vi "acquisitionZProjection.vi"(1 "axis (z)":u16(ring)=2 items=["x", "y", "z"], 2 "z stack":u16[][][](array[numeric])) -> (0 "projected img":u32[][](array[numeric]))   [LabVIEW 2017]
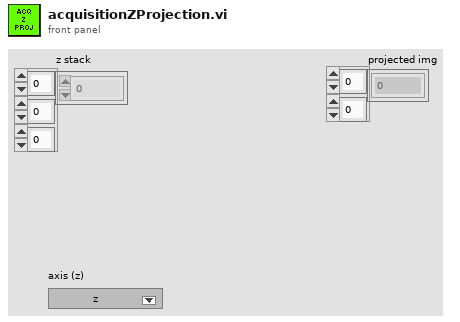
[diagram p1: front panel]
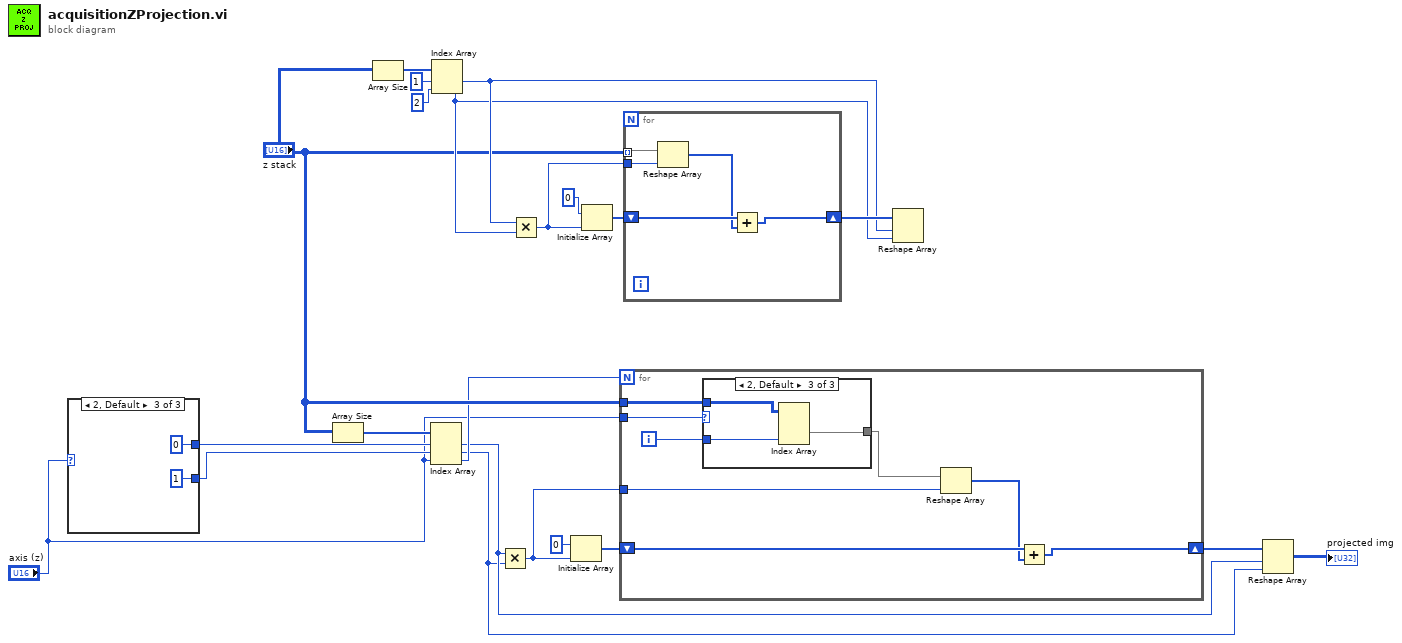
[diagram p0: block diagram]
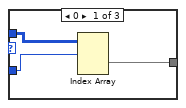
[diagram p2: hidden frame]
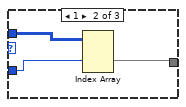
[diagram p3: hidden frame]
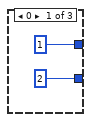
[diagram p4: hidden frame]
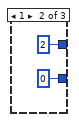
[diagram p5: hidden frame]
diagram:
  n1 = case shown="2, Default" "axis (z)" {
    tunnel: [1 2 0] -> w12
    tunnel: [2 0 1] -> w11
    frame 0 {
    }
    frame 1 {
    }
    frame 2, Default {
    }
  }
  n2 = Array Size(array="z stack") -> (size(s)=w13:i32[])
  n3 = Array Size(array="z stack") -> (size(s)=w22:i32[])
  n4 = Index Array(array=w13, index #1=w12, index #2=w11, index #3="axis (z)") -> (element #1=w3:i32, element #2=w2:i32, element #3=w8:i32)
  n5 = Index Array(array=w22, index #1=1 ("index"), index #2=2 ("index")) -> (element #1=w15:i32, element #2=w14:i32)
  n6 = Multiply(x=w3, y=w2) -> (x*y=w5:i32)
  n7 = Multiply(x=w15, y=w14) -> (x*y=w17:i32)
  n8 = Initialize Array(u32 0 ("element"), w5) -> (w6:u32[])
  n9 = Initialize Array(u32 0 ("element"), w17) -> (w18:u32[])
  n10 = for {
    N: w8 -> [_]
    tunnel: "z stack" -> [w36]
    tunnel: "axis (z)" -> [w35]
    shift-right: [w29] -> w4
    shift-left: w6 -> [w33]
    tunnel: w5 -> [w31]
    i -> [w34]
    n11 = case shown="2, Default" w35 {
      tunnel: w36 -> [w39 w42 w44]
      tunnel: w34 -> [w38 w41 w45]
      tunnel: [w37 w40 w43] -> w32
      frame 0 {
        n12 = Index Array(array=w39, index (dim 0)=w38) -> (element=w37:u16[][])  [unwired: 2 in]
      }
      frame 1 {
        n13 = Index Array(array=w42, index (dim 1)=w41) -> (element=w40:u16[][])  [unwired: 2 in]
      }
      frame 2, Default {
        n14 = Index Array(array=w44, index (dim 2)=w45) -> (element=w43:u16[][])  [unwired: 2 in]
      }
    }
    n15 = Reshape Array(w32, w31) -> (w30:u16[])
    n16 = Add(x=w33, y=w30) -> (x+y=w29:u32[])
  }
  n17 = for {
    shift-right: [w46] -> w16
    shift-left: w18 -> [w48]
    tunnel: "z stack" -> [w50] mode=indexing
    tunnel: w17 -> [w49]
    n18 = Reshape Array(w50, w49) -> (w47:u16[])
    n19 = Add(x=w48, y=w47) -> (x+y=w46:u32[])
  }
  n20 = Reshape Array(w16, w15, w14) -> ()  [unwired: 1 out]
  n21 = Reshape Array(w4, w3, w2) -> (→"projected img":u32[][])
